vi "TestFGVExercise.vi"() -> ()   [LabVIEW 2014]
uses:
  CLD3 FGV Mode.ctl
panel:
  out "Time over\n(Solution)":bool
  in  "Target Time (s)\n(Solution)":dbl=4.0
  in  "Timer-Mode\n(Solution)":T1
  out "Elapsed Time\n(Solution)":dbl
  out "Time over\n(Exercise)":bool
  in  "Target Time (s)\n(Exercise)":dbl=4.0
  out "Elapsed Time\n(Exercise)":dbl
  in  "Timer-Mode\n(Exercise)":T1
  in  "Stopp":bool
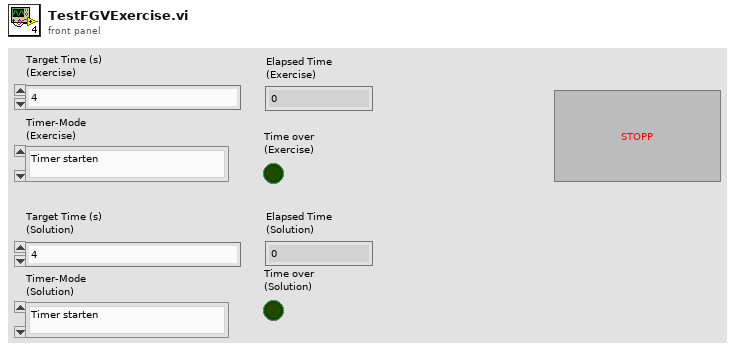
[diagram p1: front panel]
types:
  T1 = typedef "CLD3 FGV Mode.ctl" = enum16{"Timer starten", "Zeit lesen", "Anhalten", "Fortsetzen"}
  T2 = cluster{"Status":bool, "Code":i32, "Quelle":string}
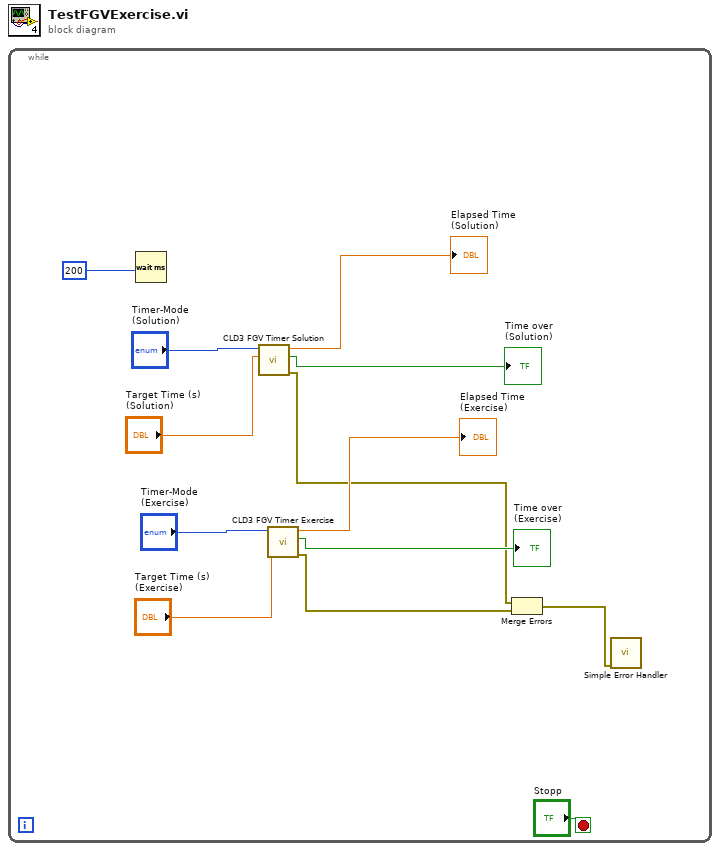
[diagram p0: block diagram]
diagram:
  n1 = while {
    stop <- "Stopp" stop-if-true
    n2 = Wait (ms)(milliseconds to wait=200) -> ()  [unwired: 1 out]
    n3 = call "CLD3 FGV Timer Solution.vi"("Zielzeit (s)"="Target Time (s)\n(Solution)", "Timer-Modus"="Timer-Mode\n(Solution)") -> ("Fehler (Ausgang)"=w3:T2, "Zeit ist verstrichen"=→"Time over\n(Solution)":bool, "Verstrichene Zeit (s,ms)"=→"Elapsed Time\n(Solution)":dbl)  [unwired: 7 in]
    n4 = call "CLD3 FGV Timer Exercise.vi"("Zielzeit (s)"="Target Time (s)\n(Exercise)", "Timer-Modus"="Timer-Mode\n(Exercise)") -> ("Fehler (Ausgang)"=w2:T2, "Zeit ist verstrichen"=→"Time over\n(Exercise)":bool, "Verstrichene Zeit (s,ms)"=→"Elapsed Time\n(Exercise)":dbl)  [unwired: 7 in]
    n5 = Merge Errors(w3, w2) -> (w1:errorcluster)
    n6 = call <vilib>:"Simple Error Handler.vi"("error in (no error)"=w1) -> ()  [unwired: 4 in, 5 out]
  }
